vi "SD Write Number.vi"(8 "error in":errorcluster, 9 "Numeric":dbl, 10 "Table Prefix":string="SmartDashboard", 11 "Name":string="Numeric") -> (0 "error out":errorcluster, 2 "Table Prefix out":string)   [LabVIEW 2017]
doc: "Write the double precision numeric data to the SmartDashboard entry -- /prefix/name."
uses:
  <vilib>/Rock Robotics/Network Tables/Field Data.ctl
  <vilib>/Rock Robotics/Network Tables/Field Type.ctl
  <vilib>/Rock Robotics/Network Tables/Sequence.ctl
  <vilib>/Rock Robotics/Network Tables/Write Value Core.vi
  <vilib>/Rock Robotics/Network Tables/Manage Dirty Field ID List.vi
  <vilib>/Rock Robotics/Network Tables/NT Globals.vi
  <vilib>/Rock Robotics/Network Tables/Update Other Clients.vi
  <vilib>/Rock Robotics/Network Tables/Build Entry Assign Buffer.vi
  <vilib>/Rock Robotics/Network Tables/Field Data Manager.vi
  <vilib>/Rock Robotics/Network Tables/Usage Statistics.vi
  <vilib>/Rock Robotics/Network Tables/Table Manager.vi
  <vilib>/Rock Robotics/Network Tables/Prepare Table Name.vi
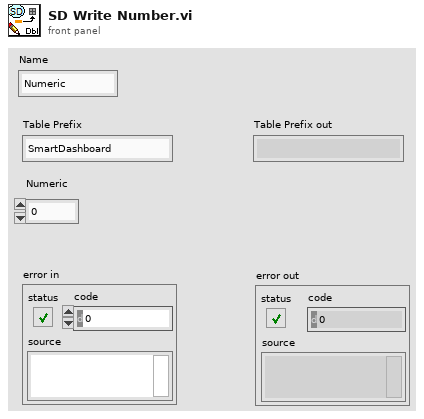
[diagram p1: front panel]
types:
  T1 = typedef "Field Data.ctl" = cluster{"Dbl":dbl, "String":string, "Type":T2, "Boolean":bool, "Sequence #":T3, "Flags":u8}
  T2 = typedef "Field Type.ctl" = enum8{"Invalid", "Bool", "Numeric", "String", "Raw", "Boolean Array", "Numeric Array", "String Array", "RPC"}
  T3 = typedef "Sequence.ctl" = u16
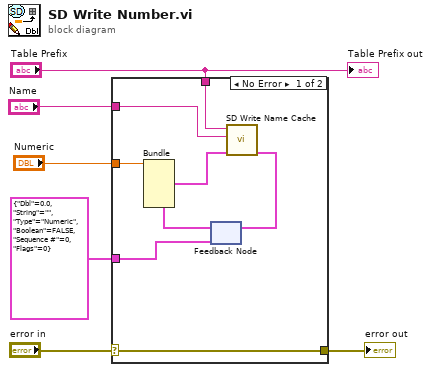
[diagram p0: block diagram]
diagram:
  n1 = case shown="No Error" "error in" {
    selector: "error in" -> [w7 w15]
    tunnel: T1 {"Dbl"=0.0, "String"="", "Type"=enum."Numeric", "Boolean"=FALSE, "Sequence #"=0, "Flags"=0} ("Field Value In") -> [w12 _]
    tunnel: "Name" -> [w10 _]
    tunnel: "Table Prefix" -> [w9 _]
    tunnel: "Numeric" -> [w8 _]
    tunnel: [w7 w15] -> w1
    frame No Error {
      n2 = feedback #1(w12) -> (w11:T1)
      n3 = Bundle(cluster=w11, "Dbl"=w8) -> (w13:T1)  [unwired: 5 in]
      n4 = call <vilib>:"SD Write Name Cache.vi"("Field Value In"=w13, "Name"=w10, "Table Prefix"=w9) -> ("Field Value Out"=w14:T1)  [unwired: 8 in]
      n5 = feedback-in #1(w14) -> ()
    }
    frame Error {
    }
  }
  "error out" <- w1
  "Table Prefix out" <- "Table Prefix"
